vi "Record Call.vi"(8 "error in (no error)":errorcluster, 11 "Mock In":refnum<class "Pure Mock.lvclass">) -> (0 "error out":errorcluster, 3 "Mock Out":refnum<class "Pure Mock.lvclass">)   [LabVIEW 2020, in "Pure Mock.lvclass"]
uses:
  Pure Mock.lvclass
  Pure Mock.lvclass/Pure Mock.ctl
  Parametric VI Call/Parametric VI Call.lvclass
  C:/git/astemes-lmock/source/Core/VI Call/VI Call.lvclass
  Core/Expectation/Expectation.lvclass
panel:
  in  "VI Name":string
  in  "Control Values":cluster{"Name":string, "Variant Data":variant}[](array[cluster])
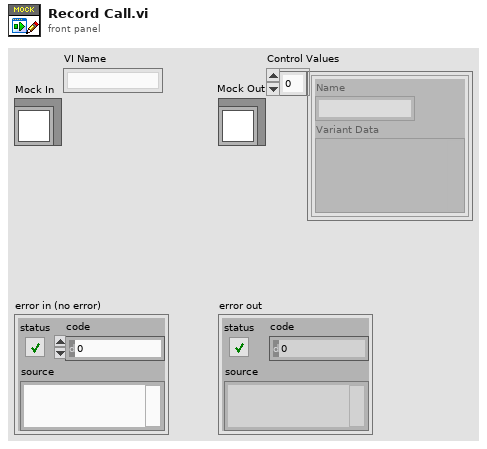
[diagram p1: front panel]
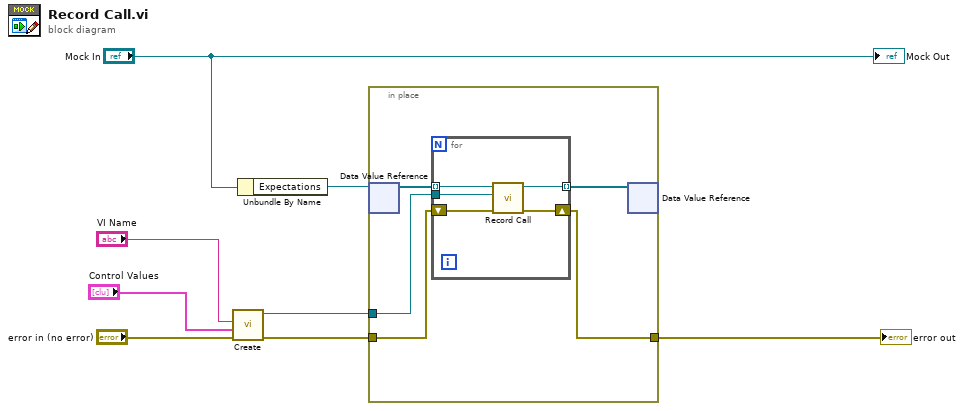
[diagram p0: block diagram]
diagram:
  n1 = call "Create.vi"("error in (no error)"="error in (no error)", "Control Values"="Control Values", "VI Name"="VI Name") -> ("error out"=w4:errorcluster, "Parametric VI Call Out"=w3:refnum<class "Parametric VI Call.lvclass">)  [unwired: 7 in]
  n2 = Unbundle By Name("Mock In") -> ("Expectations"=w8:refnum<data-value>)
  n3 = in-place {
    in-place-border: [w13] -> w6
    in-place-border: w4 -> [w12]
    in-place-border: w3 -> [w9]
    n4 = in-place-dvr #1(w8) -> (w11:refnum<class "Expectation.lvclass">[])  [unwired: 1 out]
    n5 = for {
      tunnel: w11 -> [w18] mode=indexing
      tunnel: [w17] -> w10 mode=indexing
      shift-right: [w16] -> w13
      shift-left: w12 -> [w15]
      tunnel: w9 -> [w14]
      n6 = call-dynamic "Record Call.vi"("error in (no error)"=w15, "VI Call"=w14, "Expectation in"=w18) -> ("error out"=w16:errorcluster, "Expectation out"=w17:refnum<class "Expectation.lvclass">)  [unwired: 7 in]
    }
    n7 = in-place-dvr #1(w10) -> ()  [unwired: 2 out]
  }
  "error out" <- w6
  "Mock Out" <- "Mock In"
